vi "MPExxx Self-Test.vi"(0 "VISA session":refnum<visa-resource-name>, 11 "error in (no error)":errorcluster {"code" format="%.0x"}) -> (4 "dup VISA session":refnum<visa-resource-name>, 8 "Self-Test Error":u32, 10 "Self-Test Response":string, 15 "error out":errorcluster {"code" format="%.0x"})   [LabVIEW 2012]
doc: "This VI causes the instrument to perform a self-test and returns the results. The instrument does not support a self test command."
panel:
  # "MAGNA-POWER"
  # "Electronics"
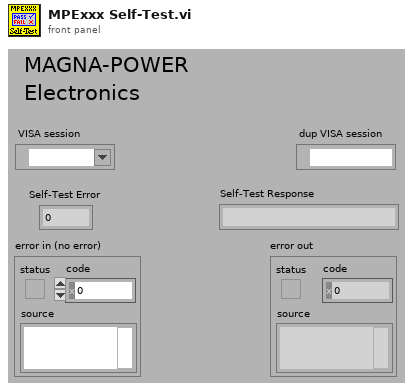
[diagram p1: front panel]
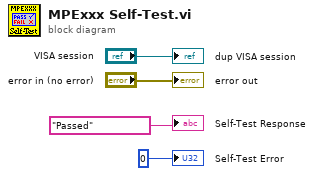
[diagram p0: block diagram]
diagram:
  "Self-Test Response" <- "Passed"
  "Self-Test Error" <- 0
  "dup VISA session" <- "VISA session"
  "error out" <- "error in (no error)"
